vi "Initialize DAQ parameters.vi"(8 "error in":errorcluster, 10 "DAQ Input Parameters(FlexRIO)":T2 {"diff_threshZ" format="%#_11g"; "proportioanl_scale Z" format="%#_15g"; "var_x" format="%#_14g"; "var_y" format="%#_14g"; "scale" format="%#_15g"; "diff_thresh" format="%#_11g"; "proportioanl_scale" format="%#_15g"}, 11 "FPGA VI Reference":T1) -> (0 "error out":errorcluster, 3 "FPGA VI Reference":T1)   [LabVIEW 2020]
uses:
  <vilib>/rvi/interface/nirviReadWriteControl/nirviReadWriteControl.xnode
  RIG-SPECIFIC FILES/FPGA Refs/FPGA Ref.ctl
  NiFpgaLv.dll
  <vilib>/Utility/error.llb/Error Cluster From Error Code.vi
  <vilib>/rvi/interface/Simulation/niFpgaSimulationCallBeginRW.vi
  <vilib>/rvi/errors/niLvFpgaAdjustHostInterfaceError.vi
  typedefs/scan_type.ctl
  Movement Correction/Typedefs/Control algorithm.ctl
  Typedefs/Controls/DAQ Input Parameters(FlexRIO).ctl
panel:
  out "Number of Trials":u16
  in  "bg_cycles":u16=40
  out "samples wait after pulse":u16=6050
  out "Samples Wait after Trigger":u16=5843
  in  "Add Cycle":bool
  in  "Slip Cycle":u32=4294967295
  # "To be integrated to one of the FGVs and read/write to file."
  # "Non-MovCor parameters"
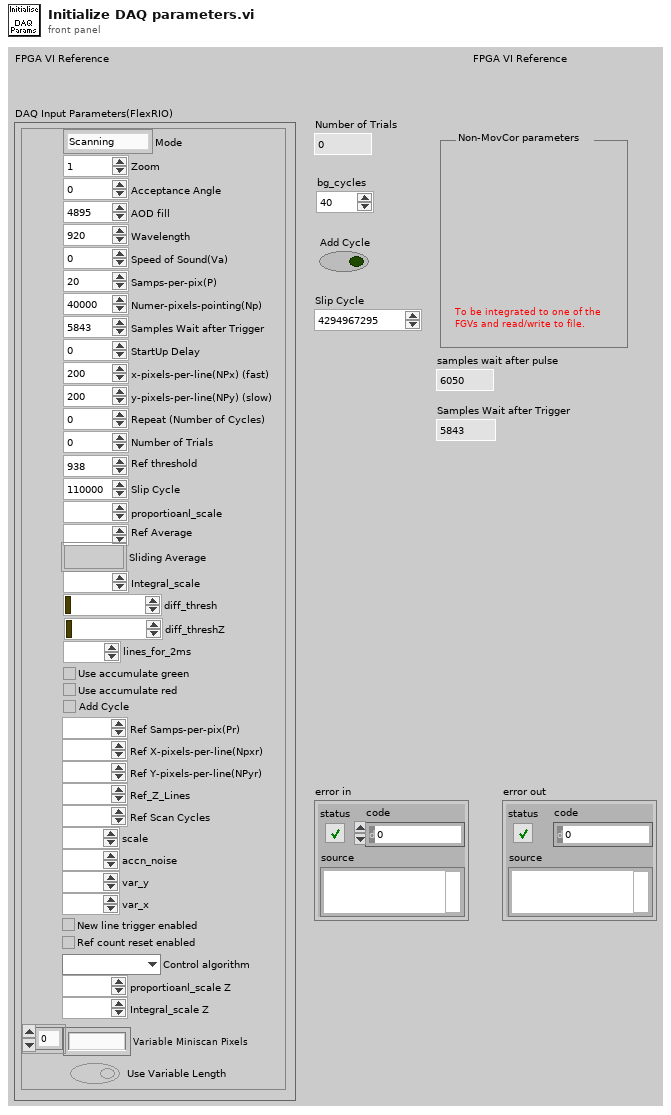
[diagram p1: front panel]
types:
  T1 = typedef "FPGA Ref.ctl" = refnum<k20>
  T2 = typedef "DAQ Input Parameters(FlexRIO).ctl" = cluster{"Mode":T3, "Zoom":i8, "Acceptance Angle":i8, "AOD fill":u16, "Wavelength":i16, "Speed of Sound(Va)":i8, "Samps-per-pix(P)":i16, "Numer-pixels-pointing(Np)":u32, "Samples Wait after Trigger":u16, "StartUp Delay":i32, "x-pixels-per-line(NPx) (fast)":u16, "y-pixels-per-line(NPy) (slow)":u16, "Repeat (Number of Cycles)":u32, "Number of Trials":u16, "Ref threshold":u16, "Slip Cycle":u32, "proportioanl_scale":fxp<+,16,2>, "Ref Average":u16, "Sliding Average":bool, "Integral_scale":fxp<+/-,16,12>, "diff_thresh":fxp<+/-,16,8>, "diff_threshZ":fxp<+/-,16,8>, "lines_for_2ms":i16, "Use accumulate green":bool, "Use accumulate red":bool, "Add Cycle":bool, "Ref Samps-per-pix(Pr)":i16, "Ref X-pixels-per-line(Npxr)":i16, "Ref Y-pixels-per-line(NPyr)":i16, "Ref_Z_Lines":i16, "Ref Scan Cycles":i32, "scale":fxp<+,16,2>, "accn_noise":fxp<+,16,16>, "var_y":fxp<+,16,4>, "var_x":fxp<+,16,4>, "New line trigger enabled":bool, "Ref count reset enabled":bool, "Control algorithm":T4, "proportioanl_scale Z":fxp<+,16,2>, "Integral_scale Z":fxp<+/-,16,12>, "Variable Miniscan Pixels":u16[], "Use Variable Length":bool}
  T3 = typedef "scan_type.ctl" = enum16{"Scanning", "Pointing", "Pointing & MC", "Scanning & MC"}
  T4 = typedef "Control algorithm.ctl" = enum16{"PID", "Kalman"}
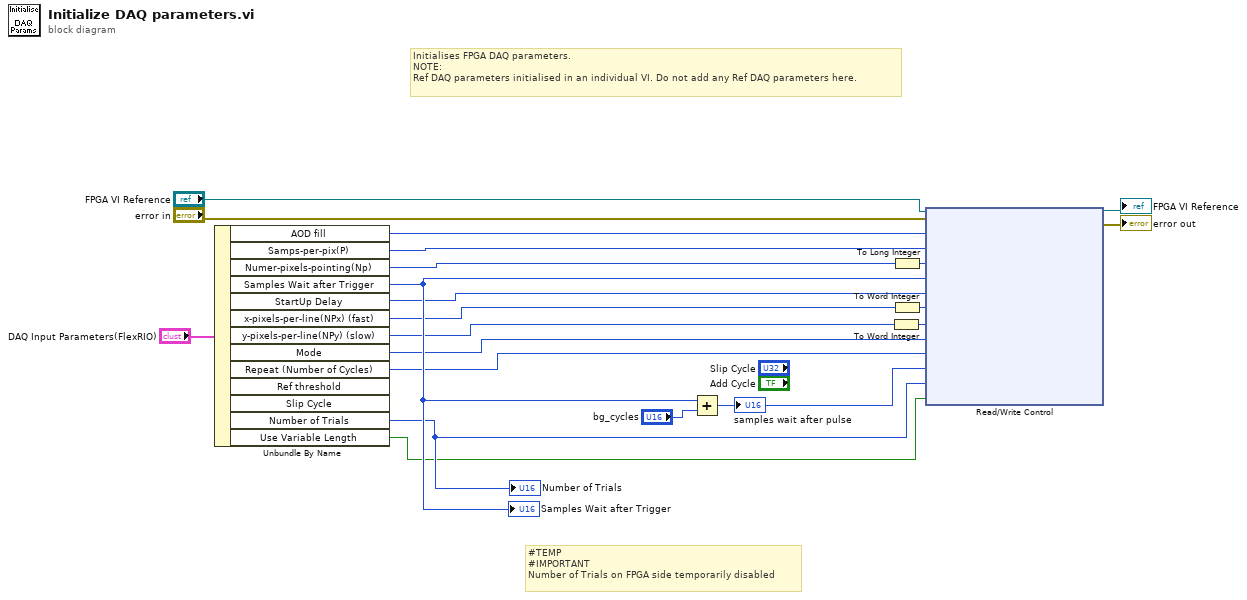
[diagram p0: block diagram]
diagram:
  # "#TEMP\n#IMPORTANT\nNumber of Trials on FPGA side temporarily disabled"
  # "Initialises FPGA DAQ parameters.\nNOTE:\nRef DAQ parameters initialised in an individual VI. Do not add any Ref DAQ parameters here."
  n1 = Unbundle By Name("DAQ Input Parameters(FlexRIO)") -> ("AOD fill"=w16:u16, "Samps-per-pix(P)"=w15:i16, "Numer-pixels-pointing(Np)"=w9:u32, "Samples Wait after Trigger"=w19:u16, "StartUp Delay"=w14:i32, "x-pixels-per-line(NPx) (fast)"=w13:u16, "y-pixels-per-line(NPy) (slow)"=w12:u16, "Mode"=w5:T3, "Repeat (Number of Cycles)"=w11:u32, "Number of Trials"=w2:u16, "Use Variable Length"=w1:bool)  [unwired: 2 out]
  "Samples Wait after Trigger" <- w19
  "Number of Trials" <- w2
  n2 = Add(x=w19, y="bg_cycles") -> (x+y=w21:u16)
  "samples wait after pulse" <- w21
  n3 = To Word Integer(number=w12) -> (16bit integer=w17:i16)
  n4 = To Long Integer(number=w9) -> (32bit integer=w10:i32)
  n5 = To Word Integer(number=w13) -> (16bit integer=w18:i16)
  n6 = xnode "Read/Write Control"("FPGA VI Reference In"="FPGA VI Reference", "error in"="error in", "AOD fill"=w16, "samps-per-pix (P)"=w15, "Number-pixels-pointing (Np)"=w10, "samples wait after trigger"=w19, "Start Up Delay"=w14, "x-pixels-per-line (Npx)"=w18, "y-pixels-per-line (Npy)"=w17, "Mode"=w5, "Repeat (Number of Cycles)"=w11, "samples wait after pulse"=w21, "trial_num_trial"=w2, "use_varailble_length"=w1) -> ("FPGA VI Reference Out"=→"FPGA VI Reference":T1, "error out"=→"error out":errorcluster)
